vi "Fault Injection Tests.vi"() -> ()   [LabVIEW 2021]
uses:
  <vilib>/Utility/Data Type/Type Definitions/Data Type.ctl
  <vilib>/numeric/Random Number (Range) DBL.vi
  <vilib>/numeric/Random Number (Range) U64.vi
  <vilib>/numeric/Random Number (Range) I64.vi
  6f91034d-b033-490f-86c8-7cba651d077e.vi
  85a68ad7-0e17-4e2b-82bf-19e681b32658.vi
  d19a7b98-5302-490e-84c7-edae248c6606.vi
  16dcf554-5919-41cd-9ee7-fb7b906522de.vi
  7f68d98e-4f2a-4a4b-aea3-2db3d99ba1d7.vi
  907ca897-7c03-4154-967b-499e17a1bb09.vi
  87041d67-1d23-4b18-b519-4f64f6546b41.vi
  07640974-a1ef-48f7-8374-010beb8d9ddb.vi
  7782772d-fc22-4723-a3c4-9704a6a2d94a.vi
  35b14a4d-3bda-42f3-a037-6612eabc0f89.vi
  fe5e3b5f-098b-42d9-80c9-5f36056fafeb.vi
  416a1639-fc69-4077-8586-0e8f4ce3b8c3.vi
  7fdcf430-8568-4010-a1dc-4fec64086319.vi
  69e68b7a-8c22-474b-b506-0cdc50535f7e.vi
  1ded0e27-309a-410f-aef7-7edceeff6ffb.vi
  09698991-96b7-4663-a1d1-3879ab0537b3.vi
  a4a60253-7054-4daa-a468-bcda414257af.vi
  bf2b3aa4-fdaf-43a2-9ad0-d8cd7fed852d.vi
  66b413c9-5705-427c-b42a-a2e1d06a8449.vi
  a5714f21-c295-44dc-8d30-f246123aad97.vi
  8ca804ec-04ce-44a7-8937-31f70e9a27f0.vi
  167317c7-3aed-471b-85dd-ea70213d9f1b.vi
  9f418bac-26d6-484c-be36-9b325f8953af.vi
  61d7fca5-f3b8-4042-be76-d188c6e759c0.vi
  5f467176-3db6-4281-9b2d-3193f550f266.vi
  c49c825b-2df1-47db-b536-2fa7e14c8900.vi
  14ff1774-db46-4b8f-a8cd-7116233270e0.vi
  bc9b0d15-7086-48db-8558-b02280d2317e.vi
  a716de72-85fe-4056-b8eb-bcc598a6c849.vi
  76fb6f51-c617-40cb-a290-2a8ad382ba34.vi
  65fd36f8-f9e4-403f-8c23-ed7a27647cd0.vi
  b370c29c-1bbc-47d1-b7f6-18f1e280d868.vi
  a04915bc-7a9d-4570-af6b-b254fede8dc1.vi
  7d414921-360e-4266-b5e0-61f5aeb1a3a2.vi
  93fe7664-50c1-46fb-8793-e3b39c135d18.vi
  fe75b306-3871-4707-afa0-fd47228b0822.vi
  e8e94303-4afb-43b7-b2cc-de7a1fce626d.vi
  24abc126-c234-46be-8ca5-29445c41d1d7.vi
  510254cf-09ec-4793-b5d9-bef02c3eaeac.vi
  <vilib>/numeric/sub_Random U32.vi
  Source/Omni-Bus/Write.vi
  Source/Omni-Bus/Support/Write/Write SGL.vi
  Source/Omni-Bus/Read.vi
  Source/Omni-Bus/Support/Read/Read SGL.vi
  Source/Fault-Injection Bus/Inject Value.vi
  Source/Fault-Injection Bus/Support/Omni-Bus/Omni-Bus Inject SGL.vi
  Source/Omni-Bus/Support/Write/Write DBL.vi
  Source/Omni-Bus/Support/Read/Read DBL.vi
  Source/Fault-Injection Bus/Support/Omni-Bus/Omni-Bus Inject DBL.vi
  Source/Omni-Bus/Support/Write/Write EXT.vi
  Source/Omni-Bus/Support/Read/Read EXT.vi
  Source/Fault-Injection Bus/Support/Omni-Bus/Omni-Bus Inject EXT.vi
  Source/Omni-Bus/Support/Write/Write CSGL.vi
  Source/Omni-Bus/Support/Read/Read CSGL.vi
  Source/Fault-Injection Bus/Support/Omni-Bus/Omni-Bus Inject CSGL.vi
  Source/Omni-Bus/Support/Write/Write CDBL.vi
  Source/Omni-Bus/Support/Read/Read CDBL.vi
  Source/Fault-Injection Bus/Support/Omni-Bus/Omni-Bus Inject CDBL.vi
  Source/Omni-Bus/Support/Write/Write CEXT.vi
  Source/Omni-Bus/Support/Read/Read CEXT.vi
  Source/Fault-Injection Bus/Support/Omni-Bus/Omni-Bus Inject CEXT.vi
  Source/Omni-Bus/Support/Write/Write I8.vi
  Source/Omni-Bus/Support/Read/Read I8.vi
  Source/Fault-Injection Bus/Support/Omni-Bus/Omni-Bus Inject I8.vi
  Source/Omni-Bus/Support/Write/Write I16.vi
  Source/Omni-Bus/Support/Read/Read I16.vi
  Source/Fault-Injection Bus/Support/Omni-Bus/Omni-Bus Inject I16.vi
  Source/Omni-Bus/Support/Write/Write I32.vi
  Source/Omni-Bus/Support/Read/Read I32.vi
  Source/Fault-Injection Bus/Support/Omni-Bus/Omni-Bus Inject I32.vi
  Source/Omni-Bus/Support/Write/Write I64.vi
  Source/Omni-Bus/Support/Read/Read I64.vi
  Source/Fault-Injection Bus/Support/Omni-Bus/Omni-Bus Inject I64.vi
  Source/Omni-Bus/Support/Write/Write U8.vi
  Source/Omni-Bus/Support/Read/Read U8.vi
  Source/Fault-Injection Bus/Support/Omni-Bus/Omni-Bus Inject U8.vi
  Source/Omni-Bus/Support/Write/Write U16.vi
  Source/Omni-Bus/Support/Read/Read U16.vi
  Source/Fault-Injection Bus/Support/Omni-Bus/Omni-Bus Inject U16.vi
  Source/Omni-Bus/Support/Write/Write U32.vi
  Source/Omni-Bus/Support/Read/Read U32.vi
  Source/Fault-Injection Bus/Support/Omni-Bus/Omni-Bus Inject U32.vi
  Source/Omni-Bus/Support/Write/Write U64.vi
  Source/Omni-Bus/Support/Read/Read U64.vi
  Source/Fault-Injection Bus/Support/Omni-Bus/Omni-Bus Inject U64.vi
  Source/Omni-Bus/Support/Write/Write Time.vi
  Source/Omni-Bus/Support/Read/Read Time.vi
  Source/Fault-Injection Bus/Support/Omni-Bus/Omni-Bus Inject Time.vi
  Source/Omni-Bus/Support/Write/Write Boolean.vi
  Source/Omni-Bus/Support/Read/Read Boolean.vi
  Source/Fault-Injection Bus/Support/Omni-Bus/Omni-Bus Inject Boolean.vi
  Source/Omni-Bus/Support/Write/Write String.vi
  Source/Fault-Injection Bus/Support/Omni-Bus/Omni-Bus Inject String.vi
  Source/Omni-Bus/Support/Write/Write Variant.vi
  Source/Omni-Bus/Support/Read/Read Variant.vi
  Source/Fault-Injection Bus/Support/Omni-Bus/Omni-Bus Inject Variant.vi
  Source/Omni-Bus/Support/Write/Write Waveform.vi
  Source/Omni-Bus/Support/Read/Read Waveform.vi
  Source/Fault-Injection Bus/Support/Omni-Bus/Omni-Bus Inject Waveform.vi
  Source/Omni-Bus/Support/Write/Write Multi SGL.vi
  Source/Omni-Bus/Support/Read/Read Multi SGL.vi
  Source/Fault-Injection Bus/Support/Omni-Bus/Omni-Bus Inject Multi SGL.vi
  Source/Omni-Bus/Support/Write/Write Multi DBL.vi
  Source/Omni-Bus/Support/Read/Read Multi DBL.vi
  Source/Fault-Injection Bus/Support/Omni-Bus/Omni-Bus Inject Multi DBL.vi
  Source/Omni-Bus/Support/Write/Write Multi EXT.vi
  Source/Omni-Bus/Support/Read/Read Multi EXT.vi
  Source/Fault-Injection Bus/Support/Omni-Bus/Omni-Bus Inject Multi EXT.vi
  Source/Omni-Bus/Support/Write/Write Multi CSGL.vi
  Source/Omni-Bus/Support/Read/Read Multi CSGL.vi
  Source/Fault-Injection Bus/Support/Omni-Bus/Omni-Bus Inject Multi CSGL.vi
  Source/Omni-Bus/Support/Write/Write Multi CDBL.vi
  Source/Omni-Bus/Support/Read/Read Multi CDBL.vi
  Source/Fault-Injection Bus/Support/Omni-Bus/Omni-Bus Inject Multi CDBL.vi
  Source/Omni-Bus/Support/Write/Write Multi CEXT.vi
  Source/Omni-Bus/Support/Read/Read Multi CEXT.vi
  Source/Fault-Injection Bus/Support/Omni-Bus/Omni-Bus Inject Multi CEXT.vi
  Source/Omni-Bus/Support/Write/Write Multi I8.vi
  Source/Omni-Bus/Support/Read/Read Multi I8.vi
  Source/Fault-Injection Bus/Support/Omni-Bus/Omni-Bus Inject Multi I8.vi
  Source/Omni-Bus/Support/Write/Write Multi I16.vi
  Source/Omni-Bus/Support/Read/Read Multi I16.vi
  Source/Fault-Injection Bus/Support/Omni-Bus/Omni-Bus Inject Multi I16.vi
  Source/Omni-Bus/Support/Write/Write Multi I32.vi
  Source/Omni-Bus/Support/Read/Read Multi I32.vi
  Source/Fault-Injection Bus/Support/Omni-Bus/Omni-Bus Inject Multi I32.vi
  Source/Omni-Bus/Support/Write/Write Multi I64.vi
  Source/Omni-Bus/Support/Read/Read Multi I64.vi
  Source/Fault-Injection Bus/Support/Omni-Bus/Omni-Bus Inject Multi I64.vi
  Source/Omni-Bus/Support/Write/Write Multi U8.vi
  Source/Omni-Bus/Support/Read/Read Multi U8.vi
  Source/Fault-Injection Bus/Support/Omni-Bus/Omni-Bus Inject Multi U8.vi
  Source/Omni-Bus/Support/Write/Write Multi U16.vi
  Source/Omni-Bus/Support/Read/Read Multi U16.vi
  Source/Fault-Injection Bus/Support/Omni-Bus/Omni-Bus Inject Multi U16.vi
  Source/Omni-Bus/Support/Write/Write Multi U32.vi
  Source/Omni-Bus/Support/Read/Read Multi U32.vi
  Source/Fault-Injection Bus/Support/Omni-Bus/Omni-Bus Inject Multi U32.vi
  Source/Omni-Bus/Support/Write/Write Multi U64.vi
  Source/Omni-Bus/Support/Read/Read Multi U64.vi
  Source/Fault-Injection Bus/Support/Omni-Bus/Omni-Bus Inject Multi U64.vi
  Source/Omni-Bus/Support/Write/Write Multi Time.vi
  Source/Omni-Bus/Support/Read/Read Multi Time.vi
  Source/Fault-Injection Bus/Support/Omni-Bus/Omni-Bus Inject Multi Time.vi
  Source/Omni-Bus/Support/Write/Write Multi Boolean.vi
  Source/Omni-Bus/Support/Read/Read Multi Boolean.vi
  Source/Fault-Injection Bus/Support/Omni-Bus/Omni-Bus Inject Multi Boolean.vi
  Source/Omni-Bus/Support/Write/Write Multi String.vi
  Source/Omni-Bus/Support/Read/Read Multi String.vi
  Source/Fault-Injection Bus/Support/Omni-Bus/Omni-Bus Inject Multi String.vi
  Source/Omni-Bus/Support/Write/Write Multi Variant.vi
  Source/Omni-Bus/Support/Read/Read Multi Variant.vi
  Source/Fault-Injection Bus/Support/Omni-Bus/Omni-Bus Inject Multi Variant.vi
  Source/Omni-Bus/Support/Write/Write Multi Waveform.vi
  Source/Omni-Bus/Support/Read/Read Multi Waveform.vi
  Source/Fault-Injection Bus/Support/Omni-Bus/Omni-Bus Inject Multi Waveform.vi
  Source/Omni-Bus/Support/Get/Get Multi SGL.vi
  Source/Omni-Bus/Support/FindMultiVar.vi
  Source/Omni-Bus/Support/Get/Get Multi DBL.vi
  Source/Omni-Bus/Support/Get/Get Multi EXT.vi
  Source/Omni-Bus/Support/Get/Get Multi CPLX_SGL.vi
  Source/Omni-Bus/Support/Get/Get Multi CPLX_DBL.vi
  Source/Omni-Bus/Support/Get/Get Multi CPLX_EXT.vi
  Source/Omni-Bus/Support/Get/Get Multi I8.vi
  Source/Omni-Bus/Support/Get/Get Multi I16.vi
  Source/Omni-Bus/Support/Get/Get Multi I32.vi
  Source/Omni-Bus/Support/Get/Get Multi I64.vi
  Source/Omni-Bus/Support/Get/Get Multi U8.vi
  Source/Omni-Bus/Support/Get/Get Multi U16.vi
  Source/Omni-Bus/Support/Get/Get Multi U32.vi
  Source/Omni-Bus/Support/Get/Get Multi U64.vi
  Source/Omni-Bus/Support/Get/Get Multi Time.vi
  Source/Omni-Bus/Support/Get/Get Multi Boolean.vi
  Source/Omni-Bus/Support/Get/Get Multi String.vi
  Source/Omni-Bus/Support/Get/Get Multi Variant.vi
  Source/Omni-Bus/Support/Get/Get Multi Waveform.vi
  Source/Local Bus/Local Bus.lvclass
  C:/TSA/Omni-Bus/Source/Omni-Bus/Bus Access/Bus_Access.lvclass
  Source/Fault-Injection Bus/Fault-Injection Bus.lvclass
  <vilib>/TSA/Abstract Data Classes/Abs_Types/Single Float/Abs_Single Float.lvclass
  C:/Program Files (x86)/National Instruments/LabVIEW 2021/vi.lib/TSA/Abstract Data Classes/Abs_Types/Type/Abs_Type.lvclass
  Source/Fault-Injection Bus/Support/Value Type/SGL/Fault-Injection_SGL.lvclass
  <vilib>/TSA/Abstract Data Classes/Abs_Types/Double Float/Abs_Double Float.lvclass
  Source/Fault-Injection Bus/Support/Value Type/DBL/Fault-Injection_DBL.lvclass
  <vilib>/TSA/Abstract Data Classes/Abs_Types/Extended Float/Abs_Extended Float.lvclass
  Source/Fault-Injection Bus/Support/Value Type/EXT/Fault-Injection_EXT.lvclass
  <vilib>/TSA/Abstract Data Classes/Abs_Types/Complex Single Float/Abs_Complex Single Float.lvclass
  Source/Fault-Injection Bus/Support/Value Type/CSGL/Fault-Injection_CSGL.lvclass
  <vilib>/TSA/Abstract Data Classes/Abs_Types/Complex Double Float/Abs_Complex Double Float.lvclass
  Source/Fault-Injection Bus/Support/Value Type/CDBL/Fault-Injection_CDBL.lvclass
  <vilib>/TSA/Abstract Data Classes/Abs_Types/Complex Extended Float/Abs_Complex Extended Float.lvclass
  Source/Fault-Injection Bus/Support/Value Type/CEXT/Fault-Injection_CEXT.lvclass
  <vilib>/TSA/Abstract Data Classes/Abs_Types/I8 Integer/Abs_I8 Integer.lvclass
  Source/Fault-Injection Bus/Support/Value Type/I8/Fault-Injection_I8.lvclass
  <vilib>/TSA/Abstract Data Classes/Abs_Types/I16 Integer/Abs_I16 Integer.lvclass
  Source/Fault-Injection Bus/Support/Value Type/I16/Fault-Injection_I16.lvclass
  <vilib>/TSA/Abstract Data Classes/Abs_Types/I32 Integer/Abs_I32 Integer.lvclass
  Source/Fault-Injection Bus/Support/Value Type/I32/Fault-Injection_I32.lvclass
  <vilib>/TSA/Abstract Data Classes/Abs_Types/I64 Integer/Abs_I64 Integer.lvclass
  Source/Fault-Injection Bus/Support/Value Type/I64/Fault-Injection_I64.lvclass
  <vilib>/TSA/Abstract Data Classes/Abs_Types/U8 Integer/Abs_U8 Integer.lvclass
  Source/Fault-Injection Bus/Support/Value Type/U8/Fault-Injection_U8.lvclass
  <vilib>/TSA/Abstract Data Classes/Abs_Types/U16 Integer/Abs_U16 Integer.lvclass
  Source/Fault-Injection Bus/Support/Value Type/U16/Fault-Injection_U16.lvclass
  <vilib>/TSA/Abstract Data Classes/Abs_Types/U32 Integer/Abs_U32 Integer.lvclass
  Source/Fault-Injection Bus/Support/Value Type/U32/Fault-Injection_U32.lvclass
  <vilib>/TSA/Abstract Data Classes/Abs_Types/U64 Integer/Abs_U64 Integer.lvclass
  Source/Fault-Injection Bus/Support/Value Type/Time/Fault-Injection_Time.lvclass
  <vilib>/TSA/Abstract Data Classes/Abs_Types/Boolean/Abs_Boolean.lvclass
  Source/Fault-Injection Bus/Support/Value Type/Boolean/Fault-Injection_Boolean.lvclass
  <vilib>/TSA/Abstract Data Classes/Abs_Types/String/Abs_String.lvclass
  Source/Fault-Injection Bus/Support/Value Type/STR/Fault-Injection_STR.lvclass
  <vilib>/TSA/Abstract Data Classes/Abs_Types/Variant/Abs_Variant.lvclass
  Source/Fault-Injection Bus/Support/Value Type/Variant/Fault-Injection_Variant.lvclass
  <vilib>/TSA/Abstract Data Classes/Abs_Types/Waveform/Abs_Waveform.lvclass
  Source/Fault-Injection Bus/Support/Value Type/WFM/Fault-Injection_WFM.lvclass
  Source/Fault-Injection Bus/Support/Value Type/U64/Fault-Injection_U64.lvclass
  <vilib>/TSA/Abstract Data Classes/Abs_Types/Time/Abs_Time.lvclass
  <vilib>/addons/_JKI Toolkits/Caraya/classes/Test/Define Test.vi
  Source/Local Bus/Initialise - From List.vi
  Source/Fault-Injection Bus/Initialise.vi
  Source/Omni-Bus/Support/FindVar.vi
  <vilib>/addons/_JKI Toolkits/Caraya/classes/Assert/Assert.vi
  <vilib>/addons/_JKI Toolkits/Caraya/classes/Assert/Assert Equal Value_Variant.vi
  Source/Fault-Injection Bus/Arm.vi
  <vilib>/addons/_JKI Toolkits/Caraya/classes/Assert/Assert Not Error.vi
  Source/Omni-Bus/Support/Read/Read String.vi
  Source/Omni-Bus/Omni_Bus.lvclass
  <vilib>/TSA/Abstract Data Classes/Abs_Types/Type/Abs_Type.lvclass
  <vilib>/Utility/Data Type/NI_Data Type.lvlib
  <vilib>/measure/NI_MAPro.lvlib
  <vilib>/measure/NI_MABase.lvlib
panel:
  out "error out":errorcluster
  in  "error in (no error)":errorcluster
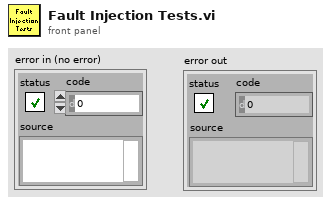
[diagram p1: front panel]
types:
  T1 = typedef "NI_Data Type.lvlib/Data Type.ctl" = enum8{"Invalid Type", "Void", "I8", "I16", "I32", "I64", "U8", "U16", "U32", "U64", "Single Float", "Double Float", "Extended Float", "Single Complex", "Double Complex", "Extended Complex", "Enum U8", "Enum U16", "Enum U32", "Enum U64", "Single Float With Unit", "Double Float With Unit", "Extended Float With Unit", "Single Complex with Unit", "Double Complex with Unit", "Extended Complex with Unit", "Boolean", "String", "Path", "Picture", "Tag", "Array", "Cluster", "Variant", "LV Variant", "Waveform", "Timestamp", "Digital Waveform", "Digital Data", "ExpressData", "Refnum", "External Data", "VI", "Poly VI", "LabVIEW Class Instance", "Fixed Point", "Set Collection", "Map Collection"}
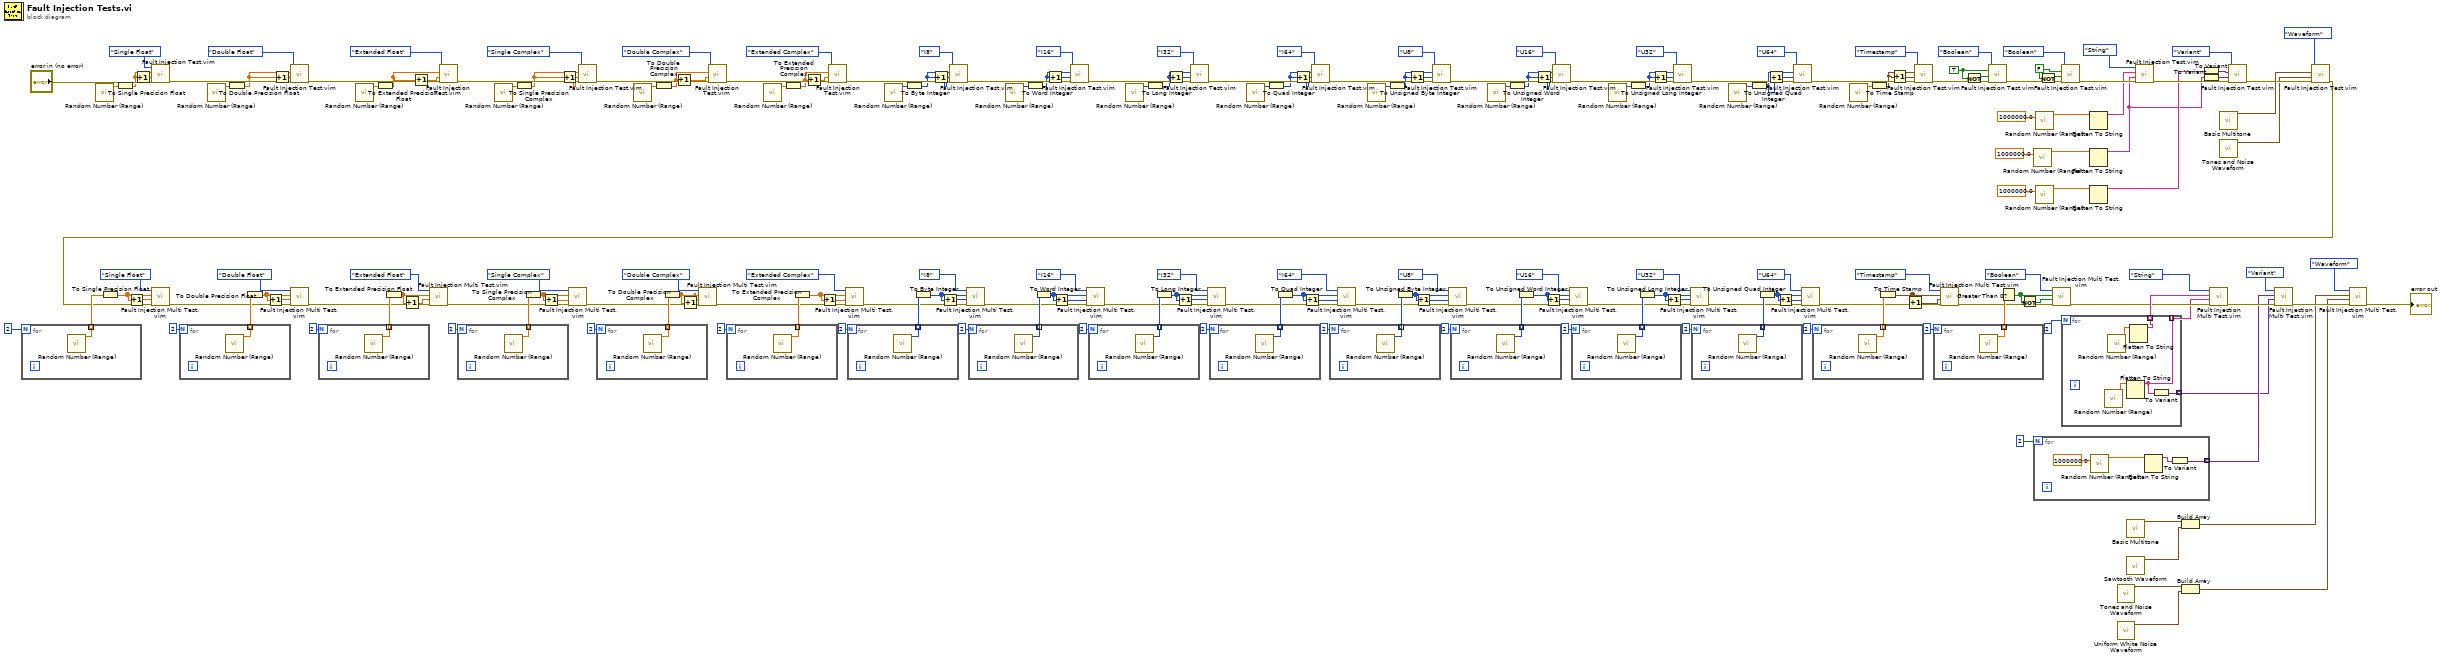
[diagram p0: block diagram]
diagram:
  w50 = FALSE
  w53 = TRUE
  n1 = for {
    N: 2 -> [_]
    tunnel: [w218] -> w155 mode=indexing
    n2 = call-poly <vilib>:"Random Number (Range).vi"() -> ("number"=w218:dbl)  [unwired: 11 in]
  }
  n3 = call-poly <vilib>:"Random Number (Range).vi"() -> ("number"=w214:dbl)  [unwired: 11 in]
  n4 = To Single Precision Float(number=w155) -> (single precision float=w45:sgl[])
  n5 = To Single Precision Float(number=w214) -> (single precision float=w82:sgl)
  n6 = Increment(x=w45) -> (x+1=w44:sgl[])
  n7 = Increment(x=w82) -> (x+1=w81:sgl)
  n8 = call "Fault Injection Test.vim"("error in (no error)"="error in (no error)", "Injected Value"=w81, "Test Value"=w82, "Type"=Data_Type."Single Float") -> ("error out"=w216:errorcluster)  [unwired: 7 in]
  n9 = for {
    N: 2 -> [_]
    tunnel: [w219] -> w153 mode=indexing
    n10 = call-poly <vilib>:"Random Number (Range).vi"() -> ("number"=w219:dbl)  [unwired: 11 in]
  }
  n11 = call-poly <vilib>:"Random Number (Range).vi"() -> ("number"=w213:dbl)  [unwired: 11 in]
  n12 = To Double Precision Float(number=w213) -> (double precision float=w1:dbl)
  n13 = To Double Precision Float(number=w153) -> (double precision float=w43:dbl[])
  n14 = Increment(x=w43) -> (x+1=w42:dbl[])
  n15 = Increment(x=w1) -> (x+1=w80:dbl)
  n16 = call "Fault Injection Test.vim"("error in (no error)"=w216, "Injected Value"=w80, "Test Value"=w1, "Type"=Data_Type."Double Float") -> ("error out"=w210:errorcluster)  [unwired: 7 in]
  n17 = for {
    N: 2 -> [_]
    tunnel: [w220] -> w147 mode=indexing
    n18 = call-poly <vilib>:"Random Number (Range).vi"() -> ("number"=w220:dbl)  [unwired: 11 in]
  }
  n19 = call-poly <vilib>:"Random Number (Range).vi"() -> ("number"=w212:dbl)  [unwired: 11 in]
  n20 = To Extended Precision Float(1:w212) -> (0:w79:ext)
  n21 = To Extended Precision Float(1:w147) -> (0:w41:ext[])
  n22 = Increment(x=w41) -> (x+1=w40:ext[])
  n23 = Increment(x=w79) -> (x+1=w78:ext)
  n24 = call "Fault Injection Test.vim"("error in (no error)"=w210, "Injected Value"=w78, "Test Value"=w79, "Type"=Data_Type."Extended Float") -> ("error out"=w207:errorcluster)  [unwired: 7 in]
  n25 = for {
    N: 2 -> [_]
    tunnel: [w221] -> w146 mode=indexing
    n26 = call-poly <vilib>:"Random Number (Range).vi"() -> ("number"=w221:dbl)  [unwired: 11 in]
  }
  n27 = call-poly <vilib>:"Random Number (Range).vi"() -> ("number"=w208:dbl)  [unwired: 11 in]
  n28 = To Single Precision Complex(1:w208) -> (0:w77:csg)
  n29 = To Single Precision Complex(1:w146) -> (0:w39:csg[])
  n30 = Increment(x=w39) -> (x+1=w38:csg[])
  n31 = Increment(x=w77) -> (x+1=w76:csg)
  n32 = call "Fault Injection Test.vim"("error in (no error)"=w207, "Injected Value"=w76, "Test Value"=w77, "Type"=Data_Type."Single Complex") -> ("error out"=w204:errorcluster)  [unwired: 7 in]
  n33 = for {
    N: 2 -> [_]
    tunnel: [w222] -> w141 mode=indexing
    n34 = call-poly <vilib>:"Random Number (Range).vi"() -> ("number"=w222:dbl)  [unwired: 11 in]
  }
  n35 = call-poly <vilib>:"Random Number (Range).vi"() -> ("number"=w206:dbl)  [unwired: 11 in]
  n36 = To Double Precision Complex(1:w206) -> (0:w75:cdb)
  n37 = To Double Precision Complex(1:w141) -> (0:w37:cdb[])
  n38 = Increment(x=w75) -> (x+1=w74:cdb)
  n39 = Increment(x=w37) -> (x+1=w36:cdb[])
  n40 = call "Fault Injection Test.vim"("error in (no error)"=w204, "Injected Value"=w74, "Test Value"=w75, "Type"=Data_Type."Double Complex") -> ("error out"=w201:errorcluster)  [unwired: 7 in]
  n41 = for {
    N: 2 -> [_]
    tunnel: [w223] -> w140 mode=indexing
    n42 = call-poly <vilib>:"Random Number (Range).vi"() -> ("number"=w223:dbl)  [unwired: 11 in]
  }
  n43 = call-poly <vilib>:"Random Number (Range).vi"() -> ("number"=w202:dbl)  [unwired: 11 in]
  n44 = To Extended Precision Complex(1:w202) -> (0:w73:cxt)
  n45 = To Extended Precision Complex(1:w140) -> (0:w35:cxt[])
  n46 = Increment(x=w73) -> (x+1=w72:cxt)
  n47 = Increment(x=w35) -> (x+1=w34:cxt[])
  n48 = call "Fault Injection Test.vim"("error in (no error)"=w201, "Injected Value"=w72, "Test Value"=w73, "Type"=Data_Type."Extended Complex") -> ("error out"=w198:errorcluster)  [unwired: 7 in]
  n49 = for {
    N: 2 -> [_]
    tunnel: [w224] -> w135 mode=indexing
    n50 = call-poly <vilib>:"Random Number (Range).vi"() -> ("number"=w224:i64)  [unwired: 11 in]
  }
  n51 = call-poly <vilib>:"Random Number (Range).vi"() -> ("number"=w200:i64)  [unwired: 11 in]
  n52 = To Byte Integer(number=w200) -> (8bit integer=w71:i8)
  n53 = To Byte Integer(number=w135) -> (8bit integer=w33:i8[])
  n54 = Increment(x=w71) -> (x+1=w70:i8)
  n55 = Increment(x=w33) -> (x+1=w32:i8[])
  n56 = call "Fault Injection Test.vim"("error in (no error)"=w198, "Injected Value"=w70, "Test Value"=w71, "Type"=Data_Type."I8") -> ("error out"=w195:errorcluster)  [unwired: 7 in]
  n57 = for {
    N: 2 -> [_]
    tunnel: [w225] -> w134 mode=indexing
    n58 = call-poly <vilib>:"Random Number (Range).vi"() -> ("number"=w225:i64)  [unwired: 11 in]
  }
  n59 = call-poly <vilib>:"Random Number (Range).vi"() -> ("number"=w196:i64)  [unwired: 11 in]
  n60 = To Word Integer(number=w196) -> (16bit integer=w68:i16)
  n61 = To Word Integer(number=w134) -> (16bit integer=w31:i16[])
  n62 = Increment(x=w68) -> (x+1=w69:i16)
  n63 = Increment(x=w31) -> (x+1=w30:i16[])
  n64 = call "Fault Injection Test.vim"("error in (no error)"=w195, "Injected Value"=w69, "Test Value"=w68, "Type"=Data_Type."I16") -> ("error out"=w192:errorcluster)  [unwired: 7 in]
  n65 = for {
    N: 2 -> [_]
    tunnel: [w226] -> w129 mode=indexing
    n66 = call-poly <vilib>:"Random Number (Range).vi"() -> ("number"=w226:i64)  [unwired: 11 in]
  }
  n67 = call-poly <vilib>:"Random Number (Range).vi"() -> ("number"=w194:i64)  [unwired: 11 in]
  n68 = To Long Integer(number=w194) -> (32bit integer=w66:i32)
  n69 = To Long Integer(number=w129) -> (32bit integer=w29:i32[])
  n70 = Increment(x=w66) -> (x+1=w67:i32)
  n71 = Increment(x=w29) -> (x+1=w28:i32[])
  n72 = call "Fault Injection Test.vim"("error in (no error)"=w192, "Injected Value"=w67, "Test Value"=w66, "Type"=Data_Type."I32") -> ("error out"=w189:errorcluster)  [unwired: 7 in]
  n73 = for {
    N: 2 -> [_]
    tunnel: [w227] -> w128 mode=indexing
    n74 = call-poly <vilib>:"Random Number (Range).vi"() -> ("number"=w227:i64)  [unwired: 11 in]
  }
  n75 = call-poly <vilib>:"Random Number (Range).vi"() -> ("number"=w190:i64)  [unwired: 11 in]
  n76 = To Quad Integer(1:w190) -> (0:w65:i64)
  n77 = To Quad Integer(1:w128) -> (0:w27:i64[])
  n78 = Increment(x=w65) -> (x+1=w64:i64)
  n79 = Increment(x=w27) -> (x+1=w26:i64[])
  n80 = call "Fault Injection Test.vim"("error in (no error)"=w189, "Injected Value"=w64, "Test Value"=w65, "Type"=Data_Type."I64") -> ("error out"=w186:errorcluster)  [unwired: 7 in]
  n81 = for {
    N: 2 -> [_]
    tunnel: [w228] -> w123 mode=indexing
    n82 = call-poly <vilib>:"Random Number (Range).vi"() -> ("number"=w228:u64)  [unwired: 11 in]
  }
  n83 = call-poly <vilib>:"Random Number (Range).vi"() -> ("number"=w188:u64)  [unwired: 11 in]
  n84 = To Unsigned Byte Integer(number=w188) -> (unsigned 8bit integer=w62:u8)
  n85 = To Unsigned Byte Integer(number=w123) -> (unsigned 8bit integer=w25:u8[])
  n86 = Increment(x=w62) -> (x+1=w63:u8)
  n87 = Increment(x=w25) -> (x+1=w24:u8[])
  n88 = call "Fault Injection Test.vim"("error in (no error)"=w186, "Injected Value"=w63, "Test Value"=w62, "Type"=Data_Type."U8") -> ("error out"=w183:errorcluster)  [unwired: 7 in]
  n89 = for {
    N: 2 -> [_]
    tunnel: [w229] -> w122 mode=indexing
    n90 = call-poly <vilib>:"Random Number (Range).vi"() -> ("number"=w229:u64)  [unwired: 11 in]
  }
  n91 = call-poly <vilib>:"Random Number (Range).vi"() -> ("number"=w184:u64)  [unwired: 11 in]
  n92 = To Unsigned Word Integer(number=w184) -> (unsigned 16bit integer=w61:u16)
  n93 = To Unsigned Word Integer(number=w122) -> (unsigned 16bit integer=w23:u16[])
  n94 = Increment(x=w61) -> (x+1=w60:u16)
  n95 = Increment(x=w23) -> (x+1=w22:u16[])
  n96 = call "Fault Injection Test.vim"("error in (no error)"=w183, "Injected Value"=w60, "Test Value"=w61, "Type"=Data_Type."U16") -> ("error out"=w180:errorcluster)  [unwired: 7 in]
  n97 = for {
    N: 2 -> [_]
    tunnel: [w230] -> w118 mode=indexing
    n98 = call-poly <vilib>:"Random Number (Range).vi"() -> ("number"=w230:u64)  [unwired: 11 in]
  }
  n99 = call-poly <vilib>:"Random Number (Range).vi"() -> ("number"=w182:u64)  [unwired: 11 in]
  n100 = To Unsigned Long Integer(number=w182) -> (unsigned 32bit integer=w59:u32)
  n101 = To Unsigned Long Integer(number=w118) -> (unsigned 32bit integer=w9:u32[])
  n102 = Increment(x=w59) -> (x+1=w58:u32)
  n103 = Increment(x=w9) -> (x+1=w10:u32[])
  n104 = call "Fault Injection Test.vim"("error in (no error)"=w180, "Injected Value"=w58, "Test Value"=w59, "Type"=Data_Type."U32") -> ("error out"=w177:errorcluster)  [unwired: 7 in]
  n105 = for {
    N: 2 -> [_]
    tunnel: [w231] -> w117 mode=indexing
    n106 = call-poly <vilib>:"Random Number (Range).vi"() -> ("number"=w231:u64)  [unwired: 11 in]
  }
  n107 = call-poly <vilib>:"Random Number (Range).vi"() -> ("number"=w178:u64)  [unwired: 11 in]
  n108 = To Unsigned Quad Integer(1:w178) -> (0:w56:u64)
  n109 = To Unsigned Quad Integer(1:w117) -> (0:w7:u64[])
  n110 = Increment(x=w56) -> (x+1=w57:u64)
  n111 = Increment(x=w7) -> (x+1=w6:u64[])
  n112 = call "Fault Injection Test.vim"("error in (no error)"=w177, "Injected Value"=w57, "Test Value"=w56, "Type"=Data_Type."U64") -> ("error out"=w173:errorcluster)  [unwired: 7 in]
  n113 = for {
    N: 2 -> [_]
    tunnel: [w232] -> w113 mode=indexing
    n114 = call-poly <vilib>:"Random Number (Range).vi"() -> ("number"=w232:dbl)  [unwired: 11 in]
  }
  n115 = call-poly <vilib>:"Random Number (Range).vi"() -> ("number"=w175:dbl)  [unwired: 11 in]
  n116 = To Time Stamp(1:w175) -> (0:w55:timestamp)
  n117 = To Time Stamp(1:w113) -> (0:w21:timestamp[])
  n118 = Increment(x=w55) -> (x+1=w54:timestamp)
  n119 = Increment(x=w21) -> (x+1=w20:timestamp[])
  n120 = call "Fault Injection Test.vim"("error in (no error)"=w173, "Injected Value"=w54, "Test Value"=w55, "Type"=Data_Type."Timestamp") -> ("error out"=w171:errorcluster)  [unwired: 7 in]
  n121 = for {
    N: 2 -> [_]
    tunnel: [w233] -> w112 mode=indexing
    n122 = call-poly <vilib>:"Random Number (Range).vi"() -> ("number"=w233:dbl)  [unwired: 11 in]
  }
  n123 = Not(x=w53) -> (.not. x?=w52:bool)
  n124 = call "Fault Injection Test.vim"("error in (no error)"=w171, "Injected Value"=w52, "Test Value"=w53, "Type"=Data_Type."Boolean") -> ("error out"=w169:errorcluster)  [unwired: 7 in]
  n125 = Greater Than 0?(x=w112) -> (x > 0?=w19:bool[])
  n126 = Not(x=w19) -> (.not. x?=w18:bool[])
  n127 = call-poly <vilib>:"Random Number (Range).vi"("upper bound (100)"=1000000.0) -> ("number"=w48:dbl)  [unwired: 10 in]
  n128 = for {
    N: 2 -> [_]
    tunnel: [w234] -> w90 mode=indexing
    n129 = call-poly <vilib>:"Random Number (Range).vi"("upper bound (100)"=1000000.0) -> ("number"=w237:dbl)  [unwired: 10 in]
    n130 = Flatten To String(anything=w237) -> (data string=w235:string)  [unwired: 3 in, 2 out]
    n131 = To Variant(anything=w235) -> (Variant=w234:variant)
  }
  n132 = call-poly <vilib>:"Random Number (Range).vi"("upper bound (100)"=1000000.0) -> ("number"=w47:dbl)  [unwired: 10 in]
  n133 = call-poly <vilib>:"Random Number (Range).vi"("upper bound (100)"=1000000.0) -> ("number"=w162:dbl)  [unwired: 10 in]
  n134 = Not(x=w50) -> (.not. x?=w51:bool)
  n135 = call "Fault Injection Test.vim"("error in (no error)"=w169, "Injected Value"=w51, "Test Value"=w50, "Type"=Data_Type."Boolean") -> ("error out"=w167:errorcluster)  [unwired: 7 in]
  n136 = for {
    N: 2 -> [_]
    tunnel: [w242] -> w107 mode=indexing
    tunnel: [w239] -> w17 mode=indexing
    tunnel: [w238] -> w16 mode=indexing
    n137 = call-poly <vilib>:"Random Number (Range).vi"() -> ("number"=w240:dbl)  [unwired: 11 in]
    n138 = call-poly <vilib>:"Random Number (Range).vi"() -> ("number"=w241:dbl)  [unwired: 11 in]
    n139 = Flatten To String(anything=w240) -> (data string=w239:string)  [unwired: 3 in, 2 out]
    n140 = Flatten To String(anything=w241) -> (data string=w242:string)  [unwired: 3 in, 2 out]
    n141 = To Variant(anything=w239) -> (Variant=w238:variant)
  }
  n142 = Flatten To String(anything=w47) -> (data string=w166:string)  [unwired: 3 in, 2 out]
  n143 = Flatten To String(anything=w48) -> (data string=w12:string)  [unwired: 3 in, 2 out]
  n144 = Flatten To String(anything=w162) -> (data string=w161:string)  [unwired: 3 in, 2 out]
  n145 = call <vilib>:"Tones and Noise Waveform.vi"() -> ("signal out"=w15:waveform(dbl))  [unwired: 10 in, 1 out]
  n146 = call <vilib>:"Uniform White Noise Waveform.vi"() -> ("signal out"=w14:waveform(dbl))  [unwired: 10 in, 1 out]
  n147 = call <vilib>:"Basic Multitone.vi"() -> ("signal out"=w85:waveform(dbl))  [unwired: 12 in, 3 out]
  n148 = call <vilib>:"Sawtooth Waveform.vi"() -> ("signal out"=w83:waveform(dbl))  [unwired: 10 in, 1 out]
  n149 = call "Fault Injection Test.vim"("error in (no error)"=w167, "Injected Value"=w12, "Test Value"=w166, "Type"=Data_Type."String") -> ("error out"=w164:errorcluster)  [unwired: 7 in]
  n150 = Build Array(w85, w83) -> (w84:waveform(dbl)[])
  n151 = Build Array(w15, w14) -> (w13:waveform(dbl)[])
  n152 = To Variant(anything=w161) -> (Variant=w4:variant)
  n153 = To Variant(anything=w12) -> (Variant=w3:variant)
  n154 = call <vilib>:"Basic Multitone.vi"() -> ("signal out"=w159:waveform(dbl))  [unwired: 12 in, 3 out]
  n155 = call <vilib>:"Tones and Noise Waveform.vi"() -> ("signal out"=w46:waveform(dbl))  [unwired: 10 in, 1 out]
  n156 = call "Fault Injection Test.vim"("error in (no error)"=w164, "Injected Value"=w3, "Test Value"=w4, "Type"=Data_Type."Variant") -> ("error out"=w158:errorcluster)  [unwired: 7 in]
  n157 = call "Fault Injection Test.vim"("error in (no error)"=w158, "Injected Value"=w46, "Test Value"=w159, "Type"=Data_Type."Waveform") -> ("error out"=w154:errorcluster)  [unwired: 7 in]
  n158 = call "Fault Injection Multi Test.vim"("error in (no error)"=w154, "Injected Value"=w44, "Test Value"=w45, "Type"=Data_Type."Single Float") -> ("error out"=w150:errorcluster)  [unwired: 7 in]
  n159 = call "Fault Injection Multi Test.vim"("error in (no error)"=w150, "Injected Value"=w42, "Test Value"=w43, "Type"=Data_Type."Double Float") -> ("error out"=w106:errorcluster)  [unwired: 7 in]
  n160 = call "Fault Injection Multi Test.vim"("error in (no error)"=w106, "Injected Value"=w40, "Test Value"=w41, "Type"=Data_Type."Extended Float") -> ("error out"=w105:errorcluster)  [unwired: 7 in]
  n161 = call "Fault Injection Multi Test.vim"("error in (no error)"=w105, "Injected Value"=w38, "Test Value"=w39, "Type"=Data_Type."Single Complex") -> ("error out"=w104:errorcluster)  [unwired: 7 in]
  n162 = call "Fault Injection Multi Test.vim"("error in (no error)"=w104, "Injected Value"=w36, "Test Value"=w37, "Type"=Data_Type."Double Complex") -> ("error out"=w103:errorcluster)  [unwired: 7 in]
  n163 = call "Fault Injection Multi Test.vim"("error in (no error)"=w103, "Injected Value"=w34, "Test Value"=w35, "Type"=Data_Type."Extended Complex") -> ("error out"=w102:errorcluster)  [unwired: 7 in]
  n164 = call "Fault Injection Multi Test.vim"("error in (no error)"=w102, "Injected Value"=w32, "Test Value"=w33, "Type"=Data_Type."I8") -> ("error out"=w101:errorcluster)  [unwired: 7 in]
  n165 = call "Fault Injection Multi Test.vim"("error in (no error)"=w101, "Injected Value"=w30, "Test Value"=w31, "Type"=Data_Type."I16") -> ("error out"=w100:errorcluster)  [unwired: 7 in]
  n166 = call "Fault Injection Multi Test.vim"("error in (no error)"=w100, "Injected Value"=w28, "Test Value"=w29, "Type"=Data_Type."I32") -> ("error out"=w99:errorcluster)  [unwired: 7 in]
  n167 = call "Fault Injection Multi Test.vim"("error in (no error)"=w99, "Injected Value"=w26, "Test Value"=w27, "Type"=Data_Type."I64") -> ("error out"=w98:errorcluster)  [unwired: 7 in]
  n168 = call "Fault Injection Multi Test.vim"("error in (no error)"=w98, "Injected Value"=w24, "Test Value"=w25, "Type"=Data_Type."U8") -> ("error out"=w97:errorcluster)  [unwired: 7 in]
  n169 = call "Fault Injection Multi Test.vim"("error in (no error)"=w97, "Injected Value"=w22, "Test Value"=w23, "Type"=Data_Type."U16") -> ("error out"=w96:errorcluster)  [unwired: 7 in]
  n170 = call "Fault Injection Multi Test.vim"("error in (no error)"=w96, "Injected Value"=w10, "Test Value"=w9, "Type"=Data_Type."U32") -> ("error out"=w95:errorcluster)  [unwired: 7 in]
  n171 = call "Fault Injection Multi Test.vim"("error in (no error)"=w95, "Injected Value"=w6, "Test Value"=w7, "Type"=Data_Type."U64") -> ("error out"=w94:errorcluster)  [unwired: 7 in]
  n172 = call "Fault Injection Multi Test.vim"("error in (no error)"=w94, "Injected Value"=w20, "Test Value"=w21, "Type"=Data_Type."Timestamp") -> ("error out"=w93:errorcluster)  [unwired: 7 in]
  n173 = call "Fault Injection Multi Test.vim"("error in (no error)"=w93, "Injected Value"=w18, "Test Value"=w19, "Type"=Data_Type."Boolean") -> ("error out"=w92:errorcluster)  [unwired: 7 in]
  n174 = call "Fault Injection Multi Test.vim"("error in (no error)"=w92, "Injected Value"=w17, "Test Value"=w107, "Type"=Data_Type."String") -> ("error out"=w91:errorcluster)  [unwired: 7 in]
  n175 = call "Fault Injection Multi Test.vim"("error in (no error)"=w91, "Injected Value"=w16, "Test Value"=w90, "Type"=Data_Type."Variant") -> ("error out"=w86:errorcluster)  [unwired: 7 in]
  n176 = call "Fault Injection Multi Test.vim"("error in (no error)"=w86, "Injected Value"=w13, "Test Value"=w84, "Type"=Data_Type."Waveform") -> ("error out"=→"error out":errorcluster)  [unwired: 7 in]
